vi "Two Shots Auto.vi"(4 "chambering speed (back)":dbl=0.7, 5 "d trim":dbl, 6 "chambering speed (front)":dbl=0.7, 7 "h trim":dbl, 9 "Height":dbl, 10 "Distance":dbl, 11 "backspin":dbl=300.0) -> ()   [LabVIEW 2011]
uses:
  <vilib>/Rock Robotics/WPI/Solenoid/WPI_SolenoidValue.ctl
  <vilib>/Rock Robotics/WPI/Solenoid/WPI_SolenoidSetEnum.vi
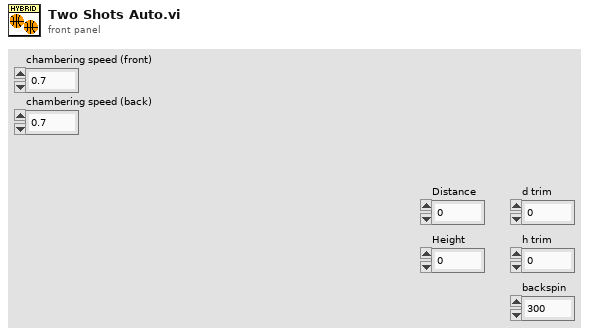
[diagram p1: front panel]
types:
  T1 = typedef "WPI_SolenoidValue.ctl" = enum16{"Off", "On", "Forward", "Reverse"}
  T2 = typedef "WPI_MotorControlDeviceRef.ctl" = cluster{"DeviceStatus":errorcluster, "Type":enum16{"PWM", "CAN"}, "PWM":cluster{"Digital Module":T3, "PWM Channel":T4, "DeadBand":T5}, "CAN":cluster{"Device Number":u8, "Control Mode":T6, "Semaphore":T7, "Max Vout":dbl}, "Invert":bool, "TransformRef":T8, "InvTransformRef":T8}
  T3 = typedef "FPGA_TypedefDigitalModule.ctl" = enum16{"Digital Module 1", "Digital Module 2"}
  T4 = typedef "FPGA_DIOPWMChannel.ctl" = enum8{"PWM 1", "PWM 2", "PWM 3", "PWM 4", "PWM 5", "PWM 6", "PWM 7", "PWM 8", "PWM 9", "PWM 10", "Invalid"}
  T5 = typedef "WPI_PWMDeadband.ctl" = cluster{"Name":string, "maxPositivePwm":i32, "minPositivePwm":i32, "centerPwm":i32, "maxNegativePwm":i32, "minNegativePwm":i32, "angularRange":u16}
  T6 = typedef "WPI_CANJaguar_ControlMode.ctl" = enum8{"Percent VBus", "Current", "Speed", "Position", "Voltage"}
  T7 = typedef "Semaphore RefNum" = refnum<k1>
  T8 = typedef "WPI_PWMTransform_ConPane.ctl" = refnum<vi>
  T9 = typedef "WPI_SolenoidDevRef.ctl" = cluster{"DevStatus":errorcluster, "Solenoid Module":T10, "Forward Solenoid Channel":T11, "Reverse Solenoid Channel":T11}
  T10 = typedef "FPGA_TypedefSolenoidModule.ctl" = enum16{"Solenoid Module 1", "Solenoid Module 2"}
  T11 = typedef "WPI_SolenoidChannel.ctl" = enum8{"Solenoid 1", "Solenoid 2", "Solenoid 3", "Solenoid 4", "Solenoid 5", "Solenoid 6", "Solenoid 7", "Solenoid 8", "Invalid"}
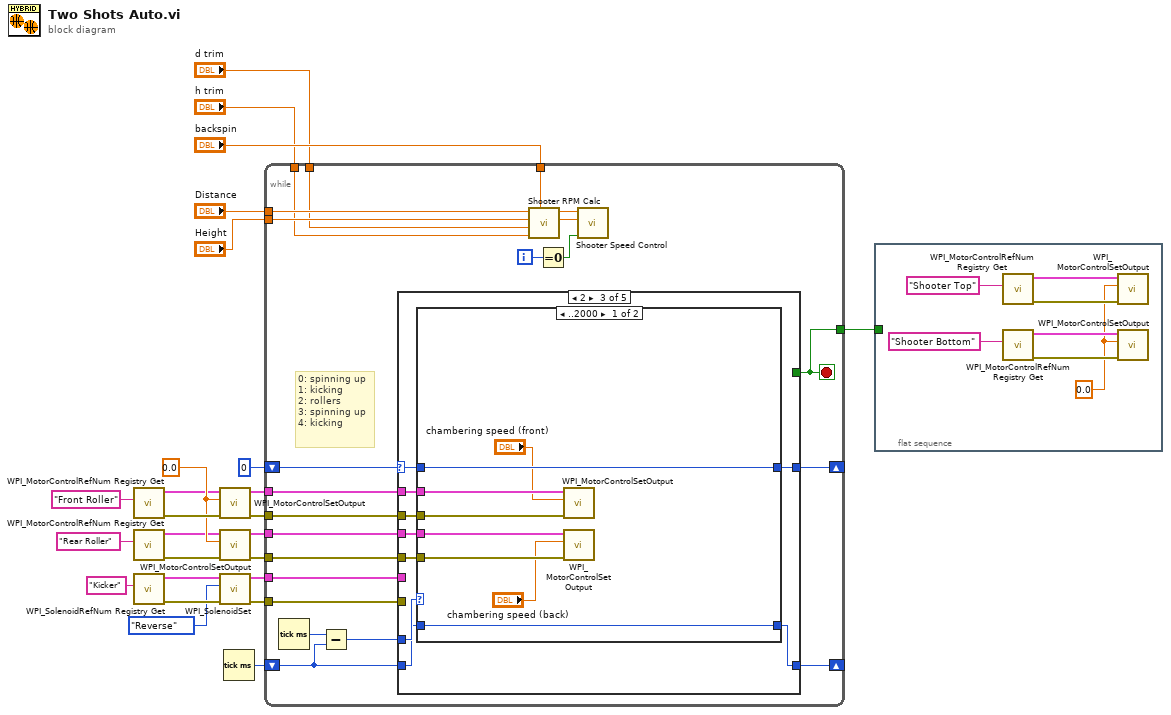
[diagram p0: block diagram]
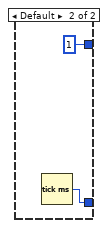
[diagram p3: hidden frame]
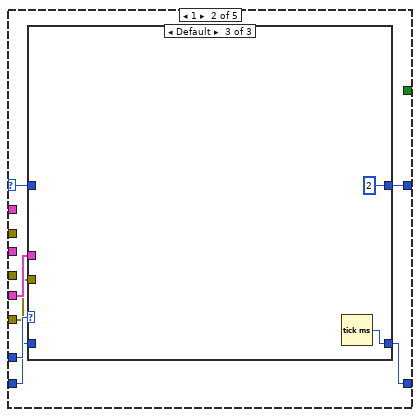
[diagram p4: hidden frame]
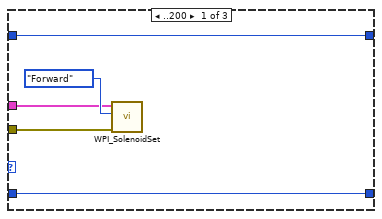
[diagram p5: hidden frame]
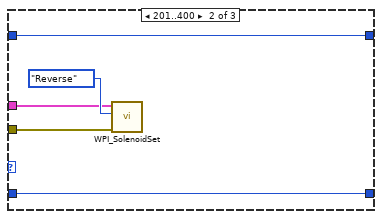
[diagram p6: hidden frame]
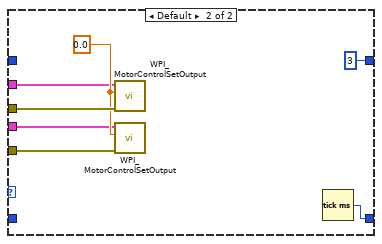
[diagram p7: hidden frame]
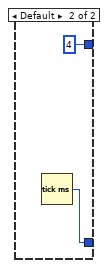
[diagram p9: hidden frame]
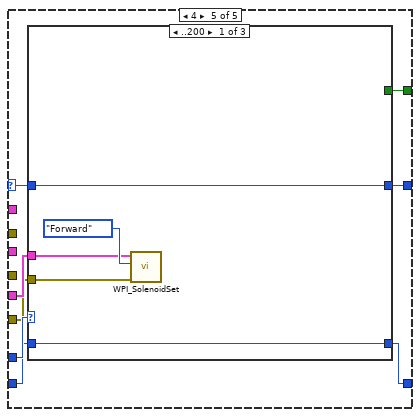
[diagram p10: hidden frame]
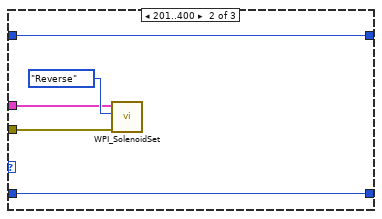
[diagram p11: hidden frame]
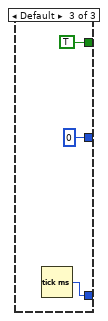
[diagram p12: hidden frame]
diagram:
  w5 = 0.0 ("RelayValue")
  n1 = call <vilib>:"WPI_MotorControlRefNum Registry Get.vi"("refnum name"="Front Roller") -> ("error out"=w15:errorcluster, "MotorControlDevRef"=w2:T2)  [unwired: 9 in]
  n2 = call <vilib>:"WPI_MotorControlRefNum Registry Get.vi"("refnum name"="Rear Roller") -> ("error out"=w7:errorcluster, "MotorControlDevRef"=w1:T2)  [unwired: 9 in]
  n3 = call <vilib>:"WPI_SolenoidRefNum Registry Get.vi"("refnum name"="Kicker") -> ("error out"=w9:errorcluster, "SolenoidDevRef"=w10:T9)  [unwired: 9 in]
  n4 = call <vilib>:"WPI_MotorControlSetOutput.vi"("error in (no error)"=w15, "Output"=w5, "MotorControlDevRef"=w2) -> ("error out"=w13:errorcluster, "MotorControlDevRef"=w14:T2)  [unwired: 7 in]
  n5 = call <vilib>:"WPI_MotorControlSetOutput.vi"("error in (no error)"=w7, "Output"=w5, "MotorControlDevRef"=w1) -> ("error out"=w3:errorcluster, "MotorControlDevRef"=w4:T2)  [unwired: 7 in]
  n6 = call-poly <vilib>:"WPI_SolenoidSet.vi"("error in (no error)"=w9, "Value"=WPI_SolenoidValue."Reverse", "SolenoidDevRef"=w10) -> ("error out"=w11:errorcluster, "SolenoidDevRef"=w12:T9)  [unwired: 7 in]
  n7 = Tick Count (ms)() -> (millisecond timer value=w23:u32)
  n8 = while {
    tunnel: "Distance" -> [w42]
    tunnel: "Height" -> [w41]
    shift-right: [w39] -> _
    shift-left: w23 -> [w38]
    shift-right: [w36] -> _
    shift-left: 0 -> [w37]
    tunnel: "backspin" -> [w35]
    tunnel: "h trim" -> [w34]
    tunnel: "d trim" -> [w33]
    tunnel: [w32] -> w18
    tunnel: w14 -> [w31]
    tunnel: w13 -> [w30]
    tunnel: w12 -> [w29]
    tunnel: w11 -> [w28]
    tunnel: w4 -> [w27]
    tunnel: w3 -> [w26]
    i -> [w45]
    stop <- w32 stop-if-true
    # "0: spinning up\n1: kicking\n2: rollers\n3: spinning up\n4: kicking"
    n9 = Tick Count (ms)() -> (millisecond timer value=w47:u32)
    n10 = Subtract(x=w47, y=w38) -> (x-y=w40:u32)
    n11 = case shown="2" w37 {
      selector: w37 -> [w48 w59 w80 w100 w112]
      tunnel: w40 -> [w52 w63 w84 w104 w116]
      tunnel: [w51 w62 w83 w103 w115] -> w39
      tunnel: w38 -> [w50 w61 w82 w102 w114]
      tunnel: [w49 w60 w81 w101 w113] -> w36
      tunnel: w29 -> [_ w58 _ _ w111]
      tunnel: w28 -> [_ w57 _ _ w110]
      tunnel: w31 -> [_ _ w79 _ _]
      tunnel: w30 -> [_ _ w78 _ _]
      tunnel: [_ _ _ _ w109] -> w32
      tunnel: w27 -> [_ _ w77 _ _]
      tunnel: w26 -> [_ _ w76 _ _]
      frame 0, Default {
        n12 = case shown="..2469" w52 {
          tunnel: [w54 w55] -> w51
          tunnel: w50 -> [w54 _]
          tunnel: [w53 1] -> w49
          tunnel: w48 -> [w53 _]
          frame ..2469 {
            # "spinning up wheels"
          }
          frame Default {
            n13 = Tick Count (ms)() -> (millisecond timer value=w55:u32)
          }
        }
      }
      frame 1 {
        n14 = case shown="Default" w63 {
          tunnel: [w68 w73 w74] -> w62
          tunnel: w61 -> [w68 w73 _]
          tunnel: [w67 w72 2] -> w60
          tunnel: w59 -> [w67 w72 _]
          tunnel: w58 -> [w65 w70 _]
          tunnel: w57 -> [w64 w69 _]
          frame ..200 {
            n15 = call-poly <vilib>:"WPI_SolenoidSet.vi"("error in (no error)"=w64, "Value"=WPI_SolenoidValue."Forward", "SolenoidDevRef"=w65) -> ()  [unwired: 7 in, 2 out]
          }
          frame 201..400 {
            n16 = call-poly <vilib>:"WPI_SolenoidSet.vi"("error in (no error)"=w69, "Value"=WPI_SolenoidValue."Reverse", "SolenoidDevRef"=w70) -> ()  [unwired: 7 in, 2 out]
          }
          frame Default {
            n17 = Tick Count (ms)() -> (millisecond timer value=w74:u32)
          }
        }
      }
      frame 2 {
        n18 = case shown="..2000" w84 {
          tunnel: [w92 w98] -> w83
          tunnel: w82 -> [w92 _]
          tunnel: [w91 3] -> w81
          tunnel: w80 -> [w91 _]
          tunnel: w79 -> [w88 w94]
          tunnel: w78 -> [w90 w97]
          tunnel: w77 -> [w87 w93]
          tunnel: w76 -> [w89 w96]
          frame ..2000 {
            n19 = call <vilib>:"WPI_MotorControlSetOutput.vi"("error in (no error)"=w90, "Output"="chambering speed (front)", "MotorControlDevRef"=w88) -> ()  [unwired: 7 in, 2 out]
            n20 = call <vilib>:"WPI_MotorControlSetOutput.vi"("error in (no error)"=w89, "Output"="chambering speed (back)", "MotorControlDevRef"=w87) -> ()  [unwired: 7 in, 2 out]
          }
          frame Default {
            w95 = 0.0 ("RelayValue")
            n21 = call <vilib>:"WPI_MotorControlSetOutput.vi"("error in (no error)"=w97, "Output"=w95, "MotorControlDevRef"=w94) -> ()  [unwired: 7 in, 2 out]
            n22 = call <vilib>:"WPI_MotorControlSetOutput.vi"("error in (no error)"=w96, "Output"=w95, "MotorControlDevRef"=w93) -> ()  [unwired: 7 in, 2 out]
            n23 = Tick Count (ms)() -> (millisecond timer value=w98:u32)
          }
        }
      }
      frame 3 {
        n24 = case shown="..500" w104 {
          tunnel: [w106 w107] -> w103
          tunnel: w102 -> [w106 _]
          tunnel: [w105 4] -> w101
          tunnel: w100 -> [w105 _]
          frame ..500 {
            # "spinning up wheels"
          }
          frame Default {
            n25 = Tick Count (ms)() -> (millisecond timer value=w107:u32)
          }
        }
      }
      frame 4 {
        n26 = case shown="..200" w116 {
          tunnel: [w121 w126 w128] -> w115
          tunnel: w114 -> [w121 w126 _]
          tunnel: [w120 w125 0] -> w113
          tunnel: w112 -> [w120 w125 _]
          tunnel: w111 -> [w118 w123 _]
          tunnel: w110 -> [w117 w122 _]
          tunnel: [_ _ TRUE] -> w109
          frame ..200 {
            n27 = call-poly <vilib>:"WPI_SolenoidSet.vi"("error in (no error)"=w117, "Value"=WPI_SolenoidValue."Forward", "SolenoidDevRef"=w118) -> ()  [unwired: 7 in, 2 out]
          }
          frame 201..400 {
            n28 = call-poly <vilib>:"WPI_SolenoidSet.vi"("error in (no error)"=w122, "Value"=WPI_SolenoidValue."Reverse", "SolenoidDevRef"=w123) -> ()  [unwired: 7 in, 2 out]
          }
          frame Default {
            n29 = Tick Count (ms)() -> (millisecond timer value=w128:u32)
          }
        }
      }
    }
    n30 = call "Shooter RPM Calc.vi"("Backspin"=w35, "Height Trim"=w34, "Distance Trim"=w33, "Height"=w41, "Distance"=w42) -> ("Bottom RPM"=w43:dbl, "Top RPM"=w44:dbl)  [unwired: 4 in, 1 out]
    n31 = Equal To 0?(x=w45) -> (x = 0?=w46:bool)
    n32 = call "Shooter Speed Control.vi"("reinitialize? (F)"=w46, "Bottom RPM"=w43, "Top RPM"=w44) -> ()  [unwired: 9 in]
  }
  n33 = flat-sequence {
    tunnel: w18 -> [_]
    frame #0 {
      w130 = 0.0 ("Output")
      n34 = call <vilib>:"WPI_MotorControlRefNum Registry Get.vi"("refnum name"="Shooter Top") -> ("error out"=w134:errorcluster, "MotorControlDevRef"=w133:T2)  [unwired: 9 in]
      n35 = call <vilib>:"WPI_MotorControlRefNum Registry Get.vi"("refnum name"="Shooter Bottom") -> ("error out"=w136:errorcluster, "MotorControlDevRef"=w135:T2)  [unwired: 9 in]
      n36 = call <vilib>:"WPI_MotorControlSetOutput.vi"("error in (no error)"=w134, "Output"=w130, "MotorControlDevRef"=w133) -> ()  [unwired: 7 in, 2 out]
      n37 = call <vilib>:"WPI_MotorControlSetOutput.vi"("error in (no error)"=w136, "Output"=w130, "MotorControlDevRef"=w135) -> ()  [unwired: 7 in, 2 out]
    }
  }
